vi "ds override minimum supported version.vi"(11 "new_version":cluster{}) -> (3 "function return":i32)   [LabVIEW 2019, in "apdm.lvlib"]
doc: "APDM_EXPORT int apdm_ds_override_minimum_supported_version(const uint64_t new_version);"
uses:
  apdm.lvlib
  Lee Lab/CP FES Walking 2018/Code/Working/LabVIEW/apdm.dll
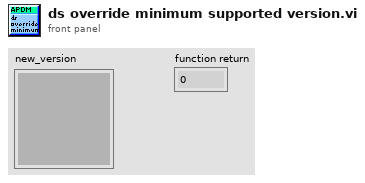
[diagram p1: front panel]
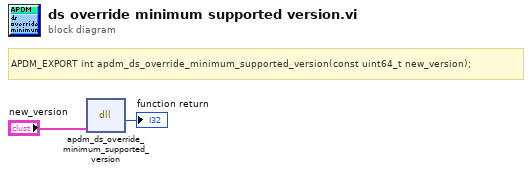
[diagram p0: block diagram]
diagram:
  # "APDM_EXPORT int apdm_ds_override_minimum_supported_version(const uint64_t new_version);"
  n1 = dll-call lib="C:/Users/jfalesi/Dropbox/Lee Lab/CP FES Walking 2018/Code/Working/LabVIEW/apdm.*" fn="apdm_ds_override_minimum_supported_version"("new_version"="new_version") -> (→"function return":i32)  [unwired: 4 in, 2 out]
